vi "InitializeObstacle.vi"(9 "Enclose obstacle? (T)":bool=TRUE, 10 "ID#":i32, 11 "Input List of UTM locations to be arranged into segments":T1[](array[typedef]) {"North" format="%#_10f"; "East" format="%#_8f"}) -> (3 "Obstacle.lvclass":refnum<class "Obstacle.lvclass">)   [LabVIEW 2013, in "Obstacle.lvclass"]
doc: "Gets an input of a list of points, outputs an obstacle. Final segment is the last and first segments. This traces the given UTM coordinates and creates line segments from each to the next, wrapping around from the last to the first. Could potentially create an obstacle like an enclosed island from this.\n\nEdited Eric Schneider, August 2014"
uses:
  Obstacle.lvclass
  Data/TypeDefs/UTM Location.ctl
  Obstacle.lvclass/Obstacle.ctl
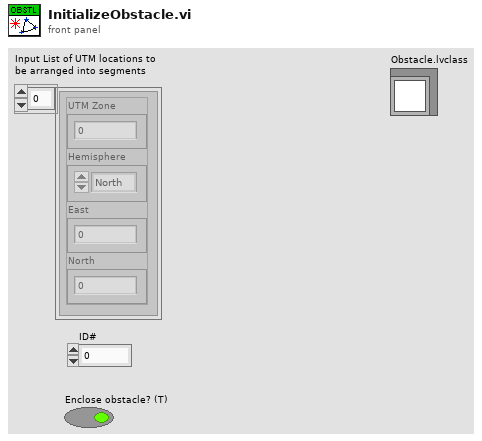
[diagram p1: front panel]
types:
  T1 = typedef "UTM Location.ctl" = cluster{"UTM Zone":dbl, "Hemisphere":enum16{"North", "South"}, "East":dbl, "North":dbl}
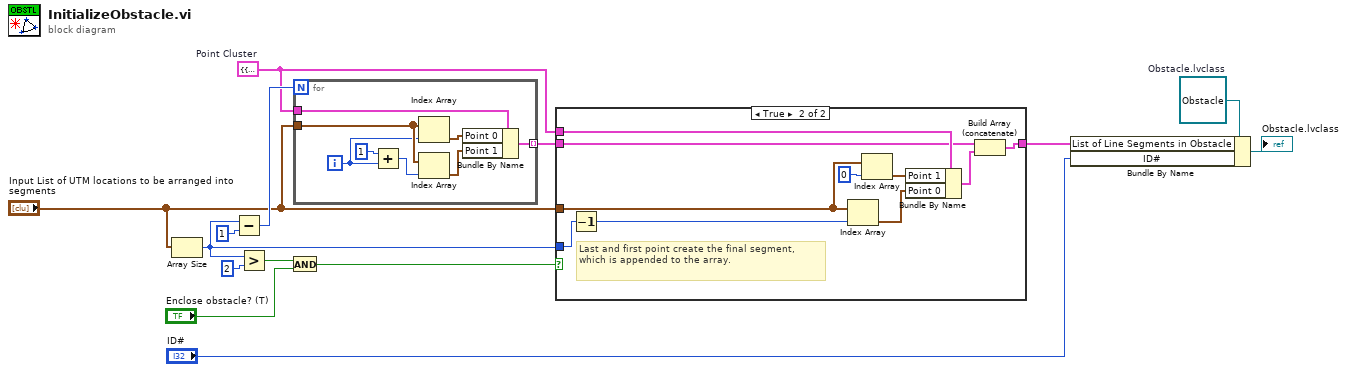
[diagram p0: block diagram]
diagram:
  w11 = refnum<class "Obstacle.lvclass"> refnum  # Obstacle.lvclass
  w10 = cluster{"Point 1":T1, "Point 0":T1} {"Point 1"={"UTM Zone"=0.0, "Hemisphere"=enum."North", "East"=0.0, "North"=0.0}, "Point 0"={"UTM Zone"=0.0, "Hemisphere"=enum."North", "East"=0.0, "North"=0.0}}  # Point Cluster
  n1 = Array Size(array="Input List of UTM locations to be arranged into segments") -> (size(s)=w6:i32)
  n2 = Subtract(x=w6, y=1) -> (x-y=w14:i32)
  n3 = Greater?(x=w6, y=2) -> (0:w4:bool)
  n4 = And(x=w4, y="Enclose obstacle? (T)") -> (x .and. y?=w2:bool)
  n5 = for {
    N: w14 -> [_]
    tunnel: "Input List of UTM locations to be arranged into segments" -> [w22]
    tunnel: [w16] -> w8 mode=indexing
    tunnel: w10 -> [w15]
    i -> [w19]
    n6 = Add(x=1, y=w19) -> (x+y=w21:i32)
    n7 = Index Array(array=w22, index=w19) -> (element=w18:T1)
    n8 = Index Array(array=w22, index=w21) -> (element=w17:T1)
    n9 = Bundle By Name(cluster=w15, "Point 0"=w18, "Point 1"=w17) -> (w16:cluster{"Point 1":T1, "Point 0":T1})
  }
  n10 = case shown="True" w2 {
    tunnel: w6 -> [_ w29]
    tunnel: w10 -> [_ w28]
    tunnel: "Input List of UTM locations to be arranged into segments" -> [_ w27]
    tunnel: w8 -> [w23 w26]
    tunnel: [w23 w24] -> w7
    frame False {
    }
    frame True {
      # "Last and first point create the final segment, which is appended to the array."
      n11 = Decrement(x=w29) -> (x-1=w33:i32)
      n12 = Index Array(array=w27, index=w33) -> (element=w32:T1)
      n13 = Index Array(array=w27, index=0) -> (element=w31:T1)
      n14 = Bundle By Name(cluster=w28, "Point 1"=w31, "Point 0"=w32) -> (w25:cluster{"Point 1":T1, "Point 0":T1})
      n15 = Build Array (concatenate)(w26, w25) -> (w24:cluster{"Point 1":T1, "Point 0":T1}[])
    }
  }
  n16 = Bundle By Name(cluster=w11, "List of Line Segments in Obstacle"=w7, "ID#"="ID#") -> (→"Obstacle.lvclass":refnum<class "Obstacle.lvclass">)
